vi "CPP-BLplotter.vi"(0 "Plot Array":cluster{dbl[], dbl[]}[](array[cluster])=[{[500.0, 500.0, 953.54, 215.0, 270.0, 320.0, 445.0, 525.0, 600.0, 675.0, 750.0, 825.0, 900.0, 960.0, 1010.0, 1060.0], [4.614524, 4.54365, 5.818368, 0.1374656, 0.6662545, 1.465458, 3.619824, 4.848976, 5.887329, 5.940571, 6.152151, 5.717487, 5.600293, 5.40069, 5.154843, 5.121789]}, {[100.0, 150.0, 215.0, 270.0, 320.0, 445.0, 525.0, 600.0, 675.0, 750.0, 825.0, 900.0, 960.0, 1010.0, 1060.0], [0.002314715, -0.00693192, 0.120417, 0.6880509, 1.519176, 3.513709, 5.065183, 6.116033, 6.096773, 5.938465, 5.593788, 5.5597, 5.387002, 5.304077, 4.887903]}] {"?" format="%.2f"; "?" format="%.2f"}, 1 "Job Directory":path=path "/G4_2_HD/Users/paulhayden/Documents/Projects/Westlakes_resolution") -> (2 "Saved Automatically?":bool, 3 "gnuplotScript":string="set term epslatex\nset output \"Plot.eps\"\nset xlabel '$Distance~(m)$'\nset ylabel '$DF~(s/m^3)\\times10^6$'\nset samples 1000\nset pointsize 1.00\nset title '$B38~Centreline~Glc$' 0, 0\nset size 0.75,0.9\n\n#set key 450, -2.5833\n unset key\nset label 1 '~~~~~~~~~~~Angle~(deg)~=~0' at -100, -2.58\nset label 2 '~~~~~~~~~~~Height~(m)~=~5' at -100, -3.27\n set xrange [0 : 500] \n# set autoscale x \n set yrange [0.10000 : 7]\n# set autoscale y \n\nplot \"B38_Centreline_Glc.dat\" index 0 using 1:2 axes x1y1 title '$File=B38R~DDD.xls$' with points 1 1, \\\n\"B38_Centreline_Glc.dat\" index 1 using 1:2 axes x1y1 title '$File=B38R~DDD~1.xls$' with points 1 3", 4 "Plot data file":path)   [LabVIEW 2012]
uses:
  Results_plotter_Global.vi
panel:
  in  "Tab Control":enum32{"Good Shit", "Boring Shit"}(tab)
  in  "Cancel Button":bool
  in  "Print Button":bool
  out "Velocity":cluster{dbl[], dbl[]}(graph)
  out "Turbulence":cluster{dbl[], dbl[]}(graph)
  in  "Plot Title":u16(ring) items=["Title String Only", "Number of Measurements", "Date::", "Profile::", "Multi Run:Start Time:", "Multi Run:Row:Type", "Multi Run:Row:Number", "Point:Time:", "Time:Stamp:", "Measuring:Instrument:Type", "Multirun:Comments:", "Run:Messages:", "Repeat::", "U_{HF}/U_{ref}::", "U_{5HP}/U_{ref}::", "TI_{HF}:%:", "TI_{U(5HP)}:%:", "Vmag_{5HP}/U_{ref}::", "V_{5HP}/U_{5HP}::", "W_{5HP}/U_{5HP}::", "U_{ref}::", "U_{HF}::", "Vmag_{5HP}::", "U_{5HP}::", "V_{5HP}::", "W_{5HP}::", "L(U):Est:(m)", "X_{5HP}:(mm):", "X_{HF}:(mm):", "Y_{5HP}:(mm):", "Y_{HF}:(mm):", "Z_{5HP}:(mm):", "Z_{HF}:(mm):", "Tau(HF)::", "Tau(5HP1)::(nose)", "Tau(5HP2)::(bottom)", "Tau(5HP3)::(top)", "Tau(5HP4)::(side)", "Tau(5HP5)::(side)", "uhf^2::", "uhf^3/(uhf^2)^1.5::", "(uhf^4/(uhf^2)^2) -3::", "HW (Uhf):Standard Error:in Mean", "HW (Uhf):Standard Error:in Variance", "HW (Uhf):Calibration:Filename", "5HP:Mode:", "5HP:ReturnType:", "Reference:Temperature:Used for Corrections", "Atmos:Pressure:Used for Corrections", "Av Analogue:Sampling:Rate", "No of:Analogue:Samples", "No Of:Measurement:Blocks", "Flow:Measurement:Time", "X:(URef):(mm)", "Y:(URef):(mm)", "Z:(URef):(mm)", "Original:Results:Filename", "Current:Data:Filename", "Current:Data File:1st Folder level", "Current:Data File:2nd Folder level", "Current:Data File:3rd Folder level", "Current:Data File:4th Folder level", "Current:File:Number", "Raw:Data:Filename", "Tunnel1 Metadata:Profile:Code", "Vmag_SD::", "U_SD::", "V_SD::", "W_SD::", "GoodFraction::"]
  in  "Filename Max length":i32=255
  out "Final Title":string="B38 Centreline Glc"
  out "Path":path
  in  "Plot Title Post Block":string
  in  "Plot Title Pre Block":string
  in  "Show Script Editor?":bool
  out "Array":string[](array[string])
  out "t":string
  # "put a load of nice controls here for ref height etc, then a button to say \"print it\" that makes and runs a gnuplot script for \nthe graphs as you have them....."
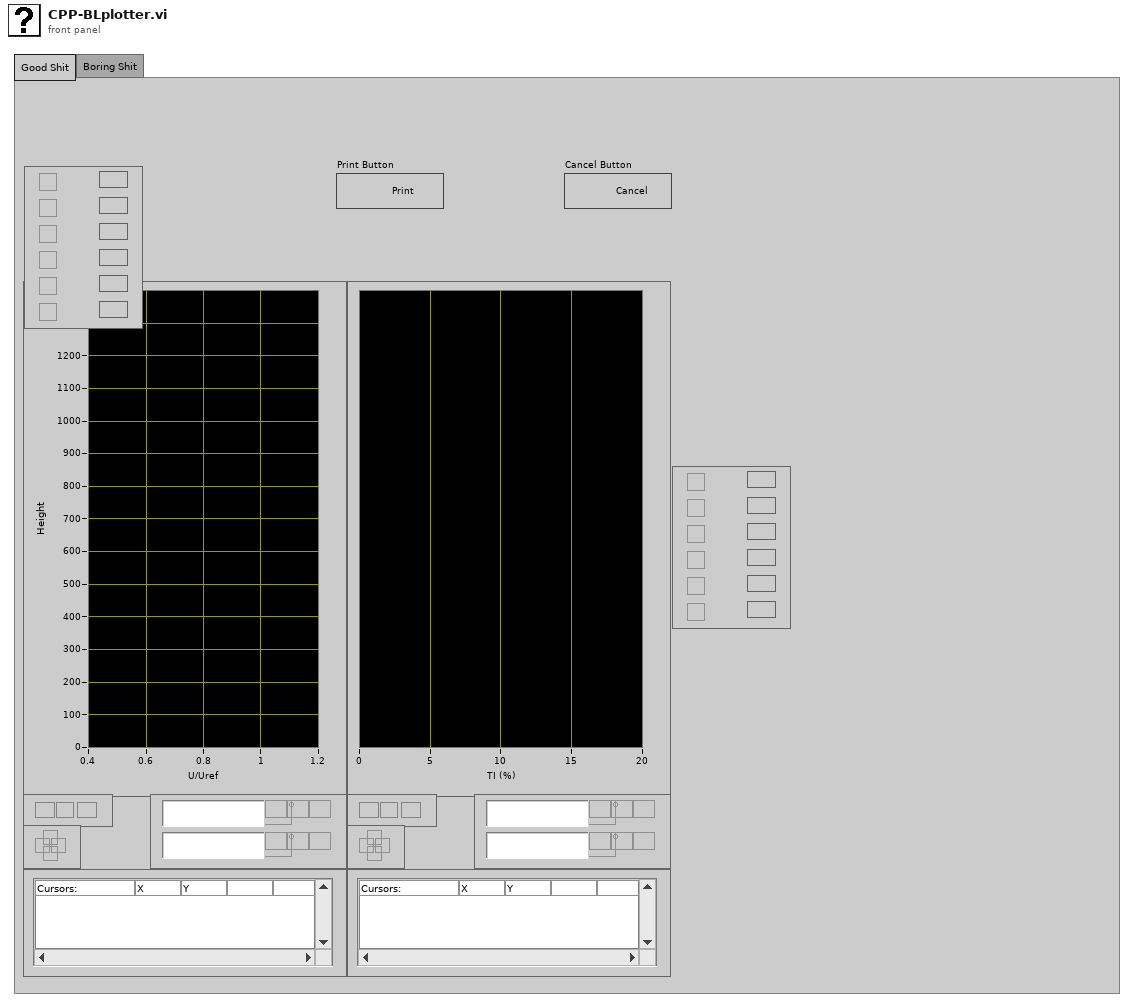
[diagram p1: front panel]
types:
  T1 = typedef "LVRangeTypeDef.ctl" = cluster{"Minimum":dbl, "Maximum":dbl, "Increment":dbl, "Minor Increment":dbl, "Start":dbl}
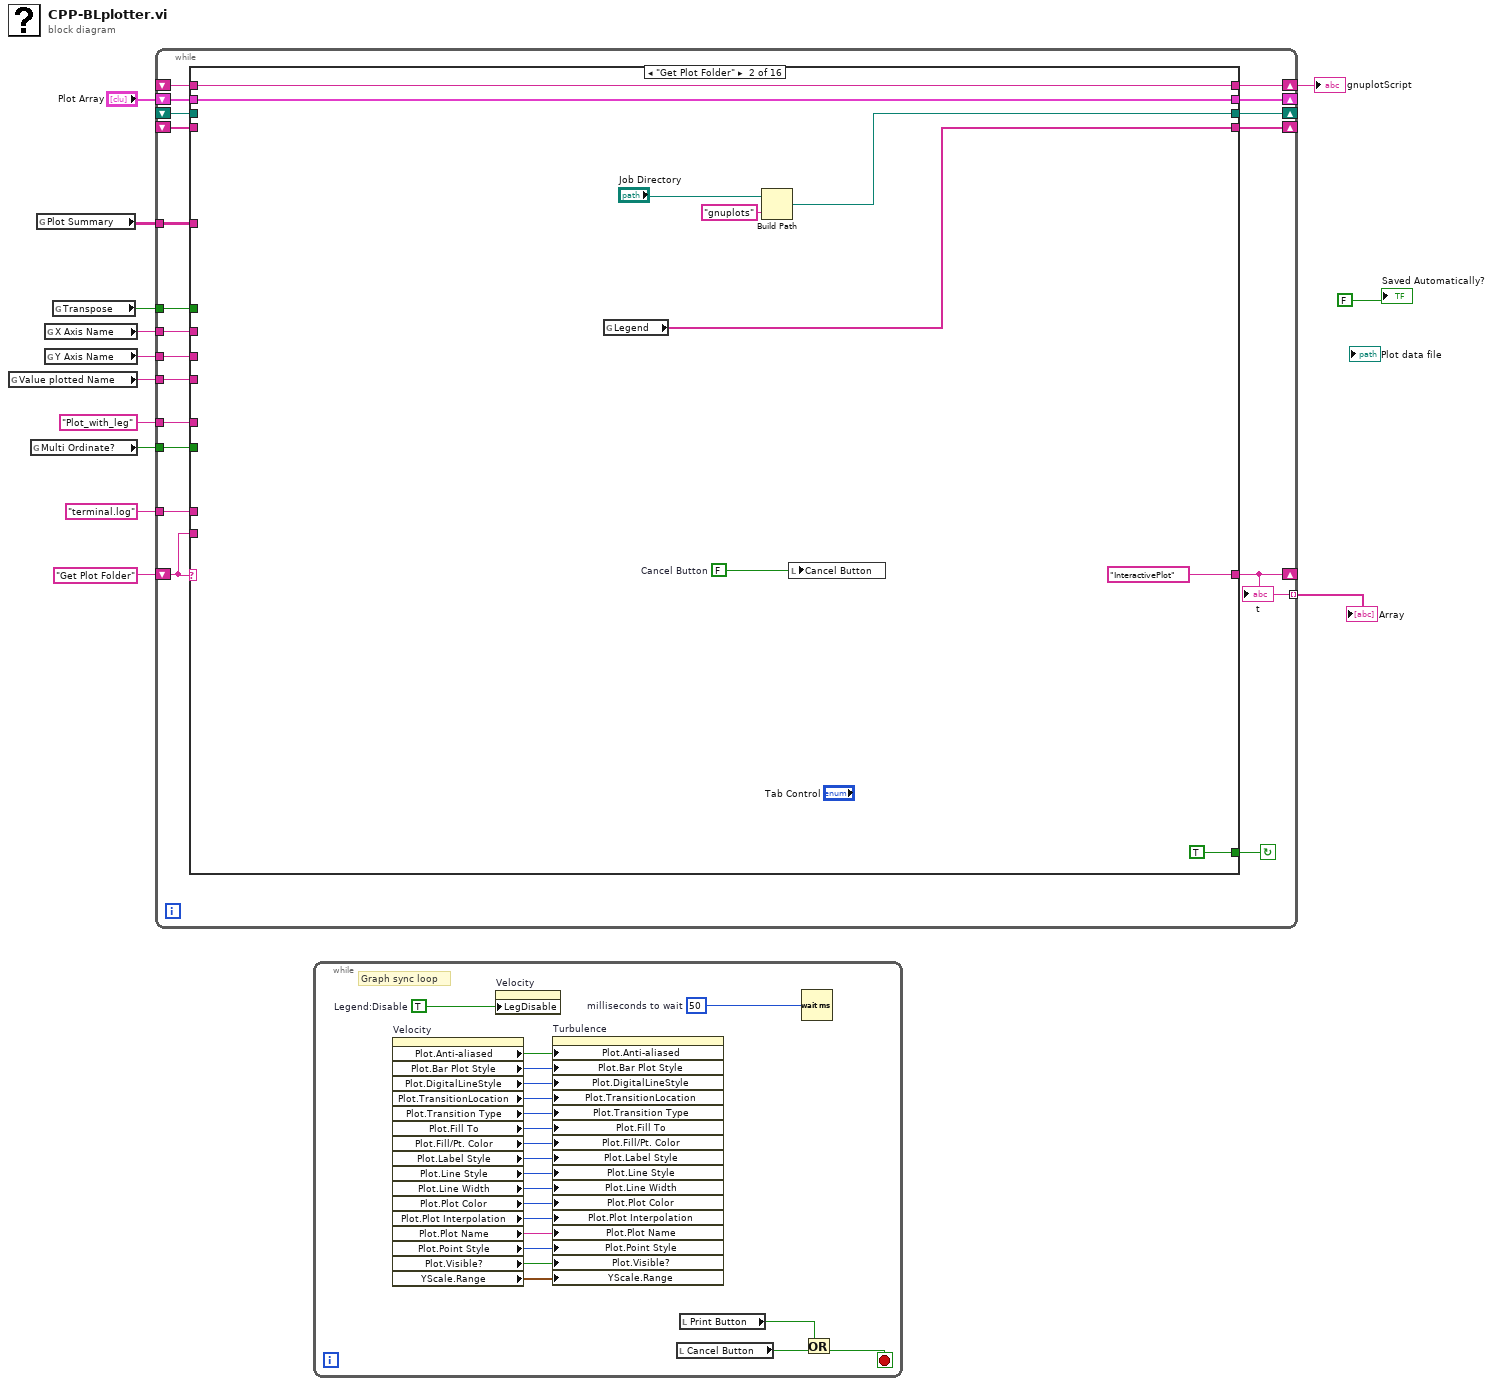
[diagram p0: block diagram]
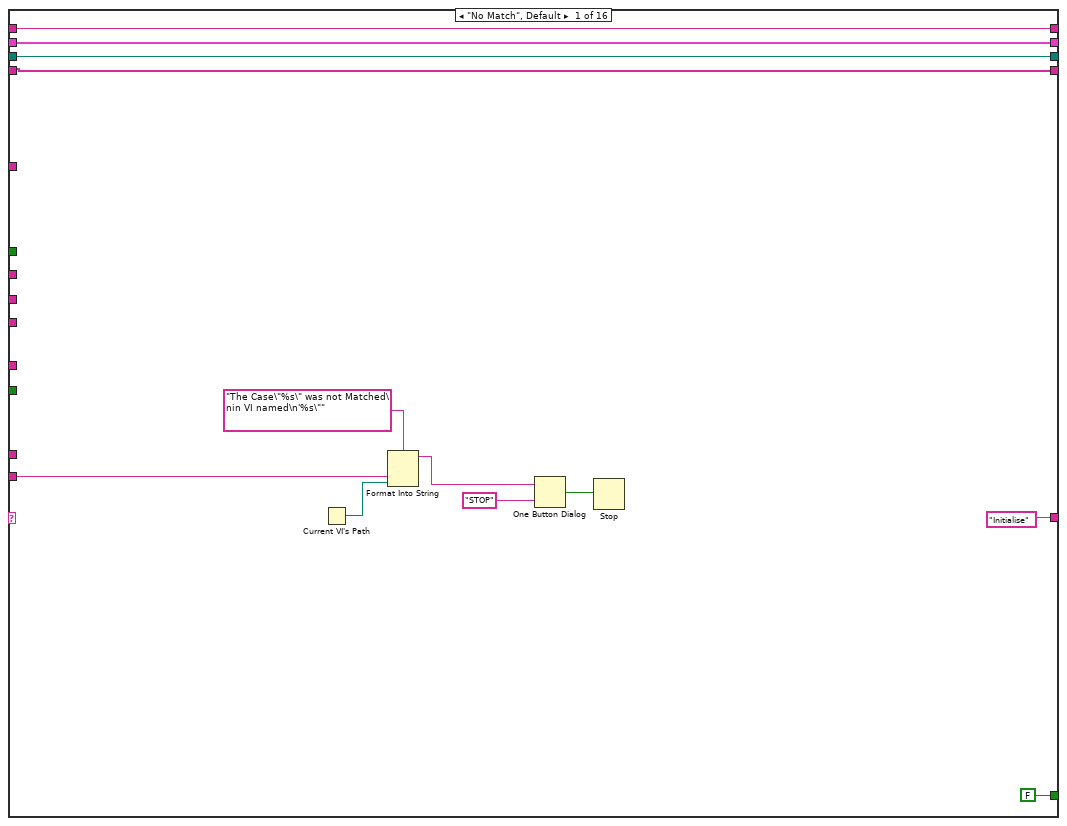
[diagram p2: hidden frame]
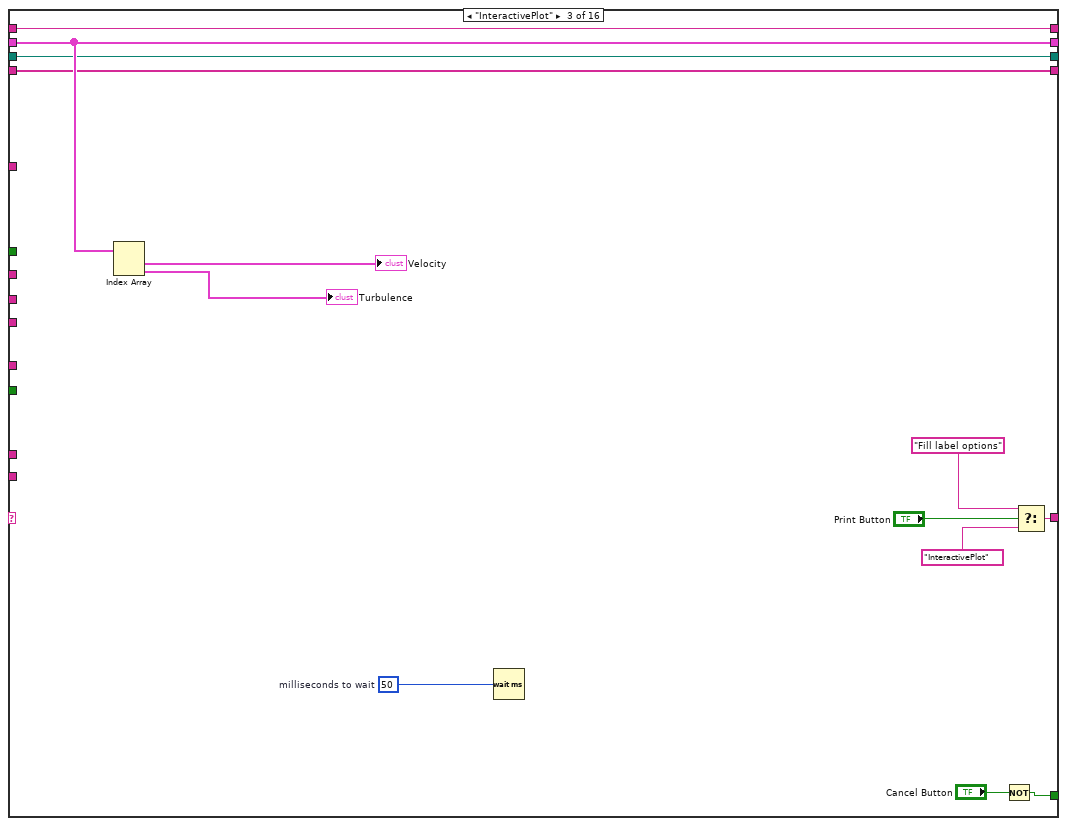
[diagram p3: hidden frame]
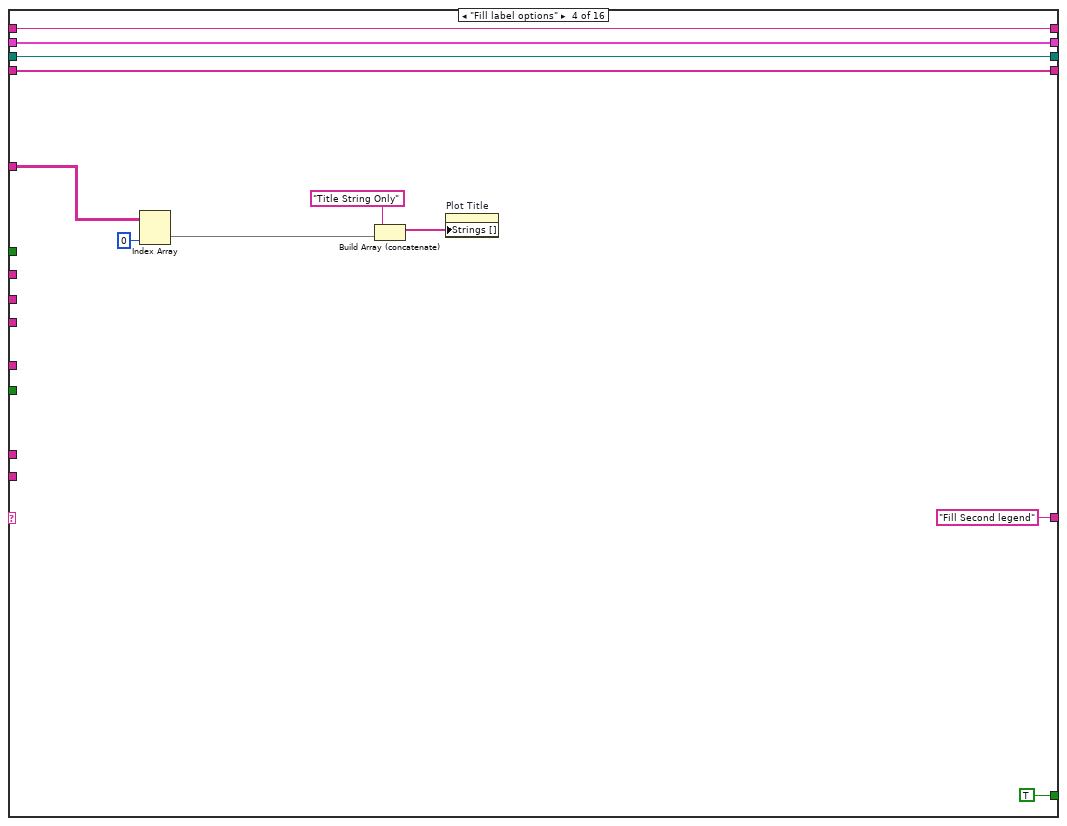
[diagram p4: hidden frame]
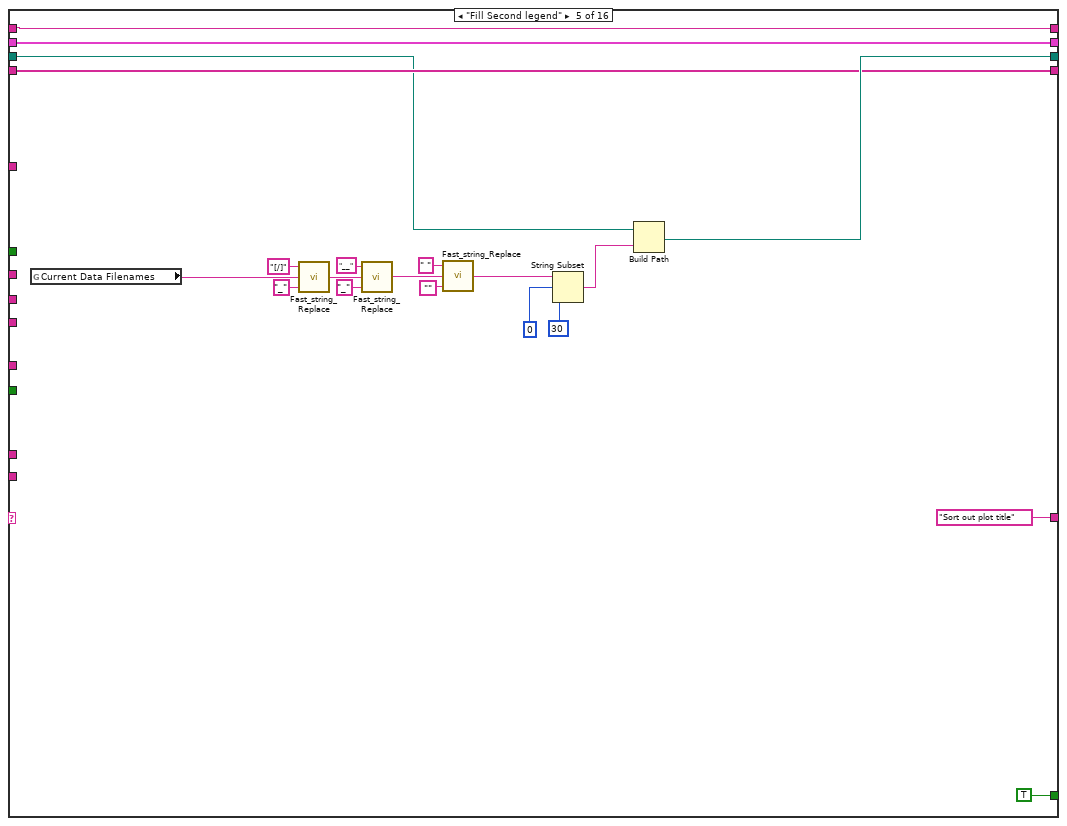
[diagram p5: hidden frame]
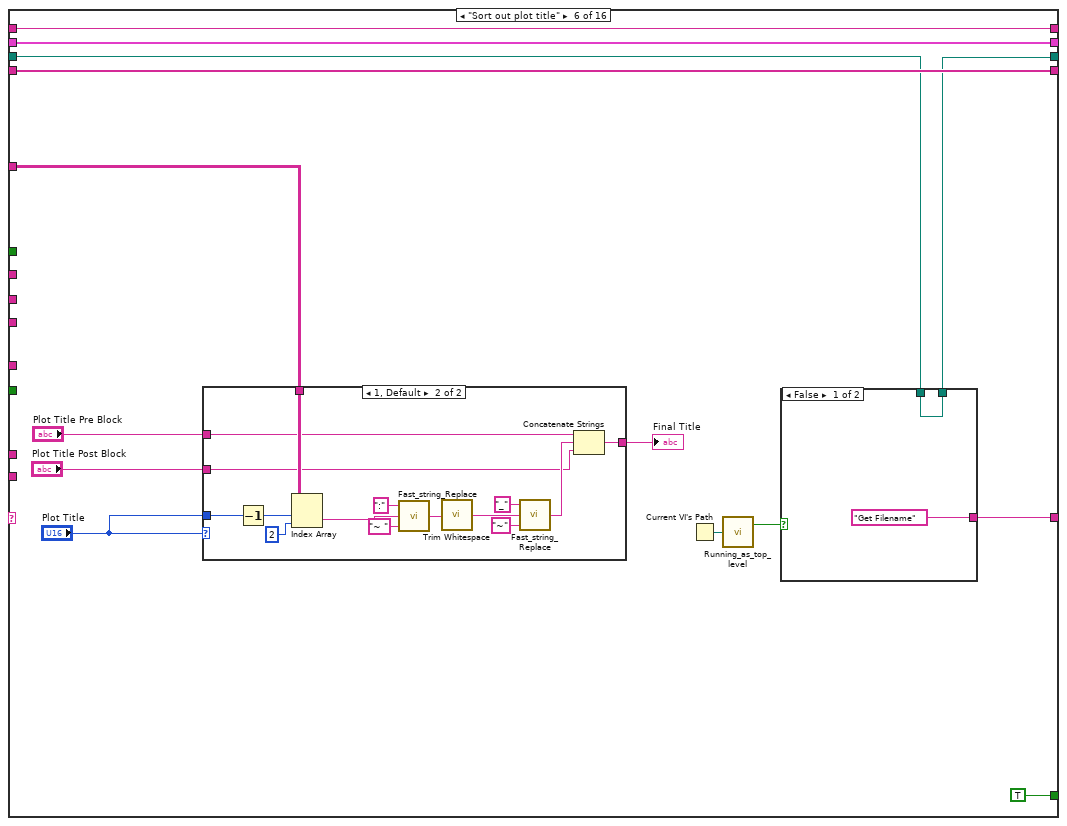
[diagram p6: hidden frame]
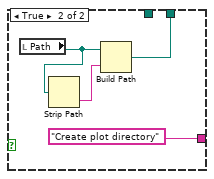
[diagram p7: hidden frame]
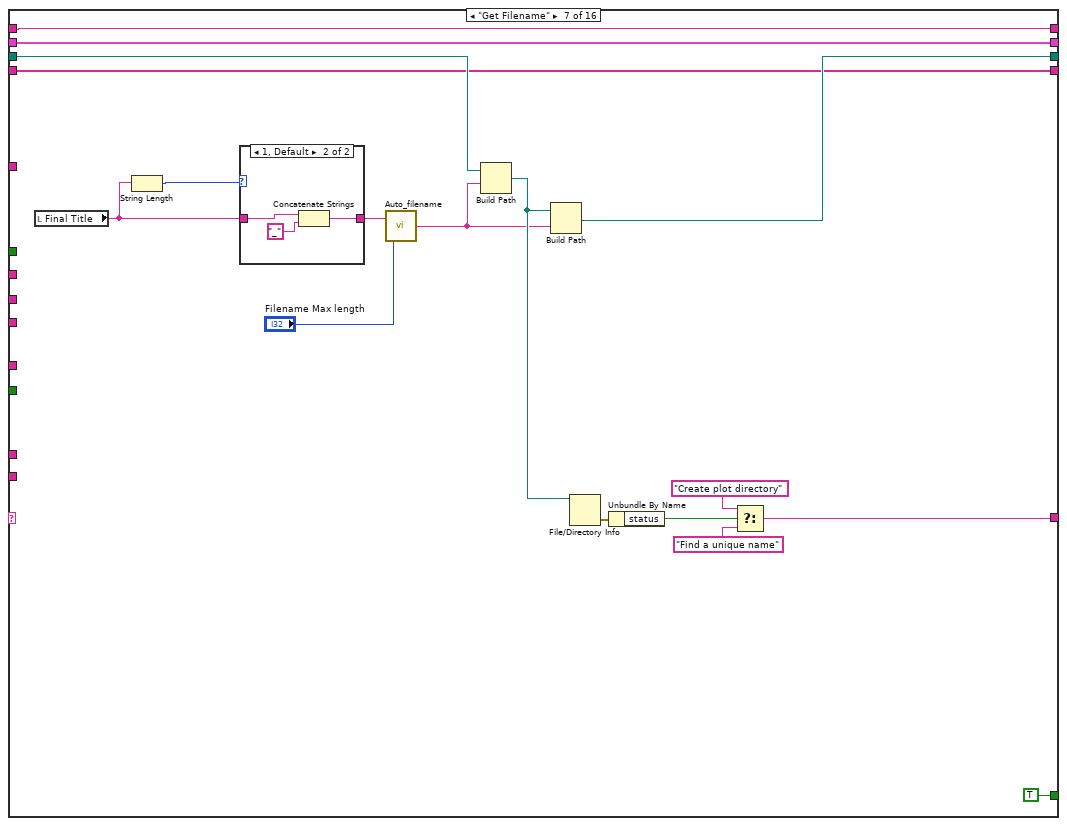
[diagram p9: hidden frame]
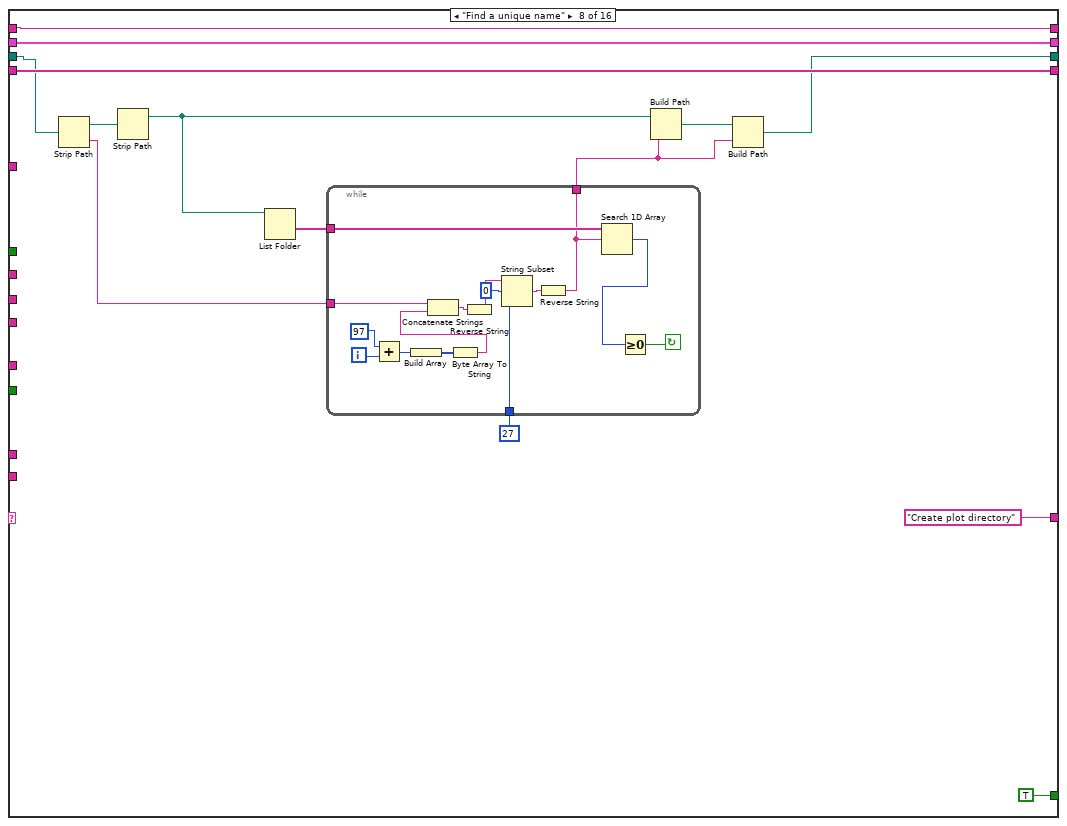
[diagram p11: hidden frame]
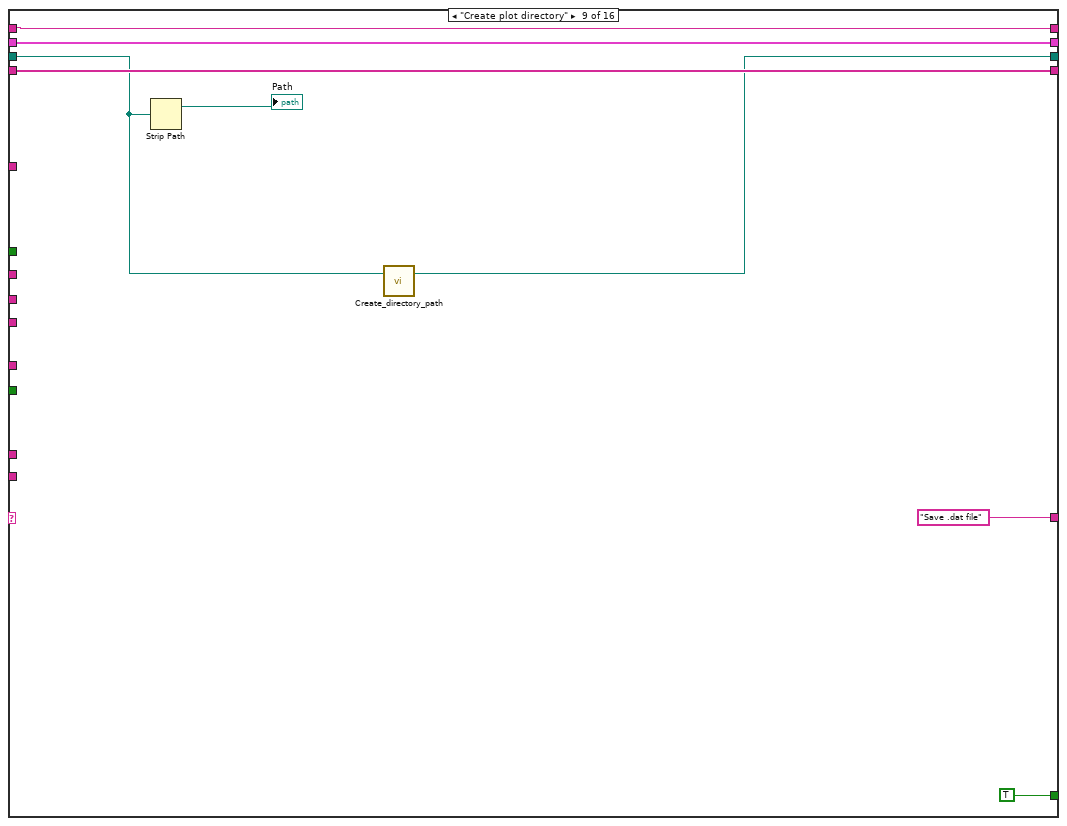
[diagram p12: hidden frame]
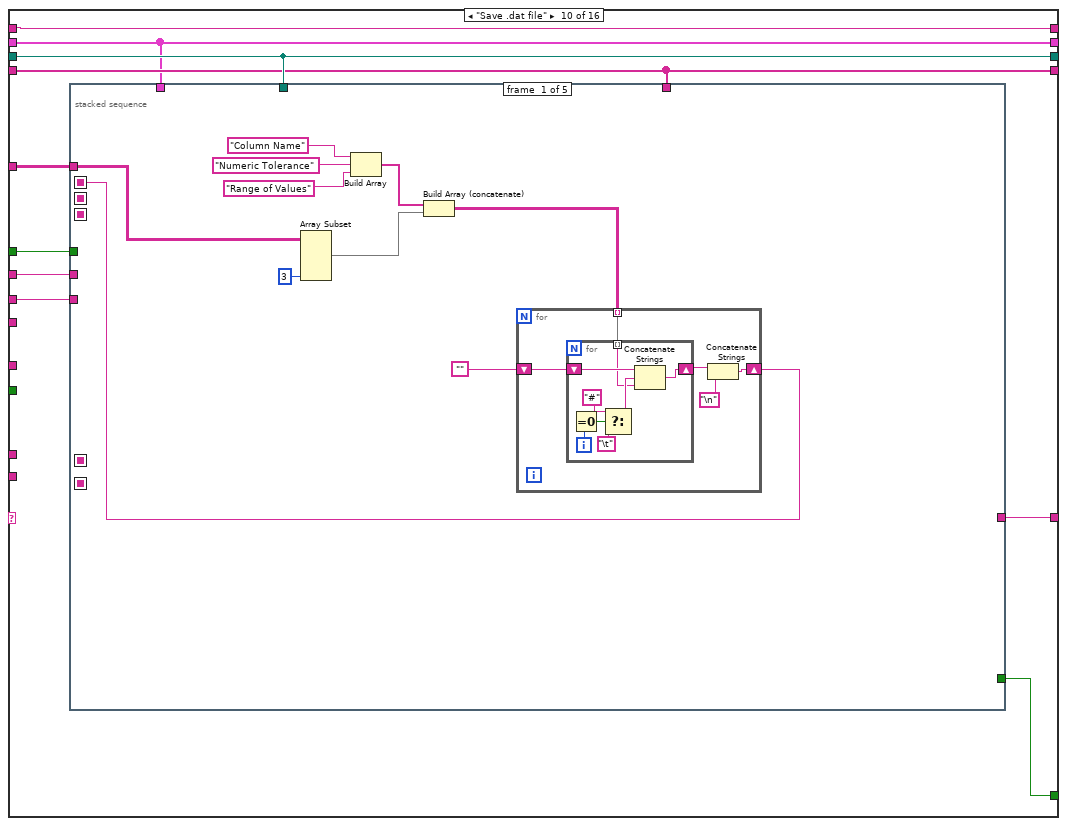
[diagram p13: hidden frame]
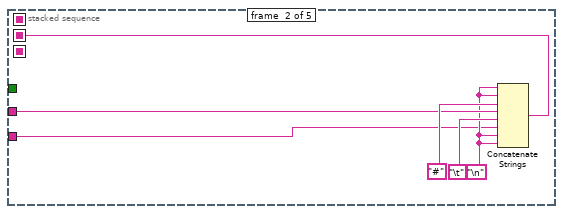
[diagram p14: hidden frame]
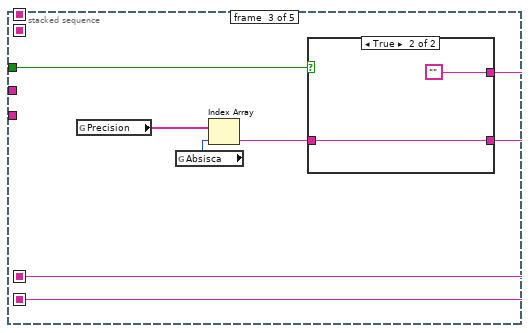
[diagram p15: hidden frame]
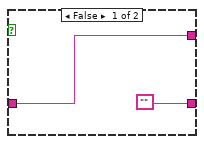
[diagram p16: hidden frame]
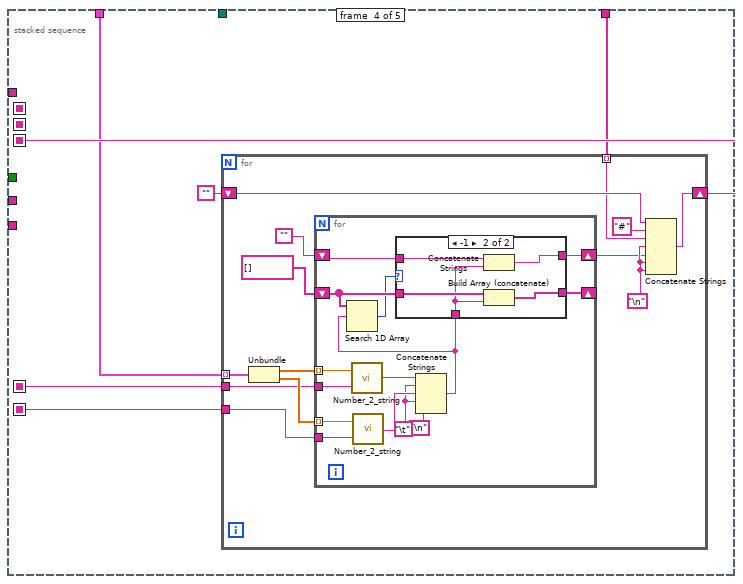
[diagram p17: hidden frame]
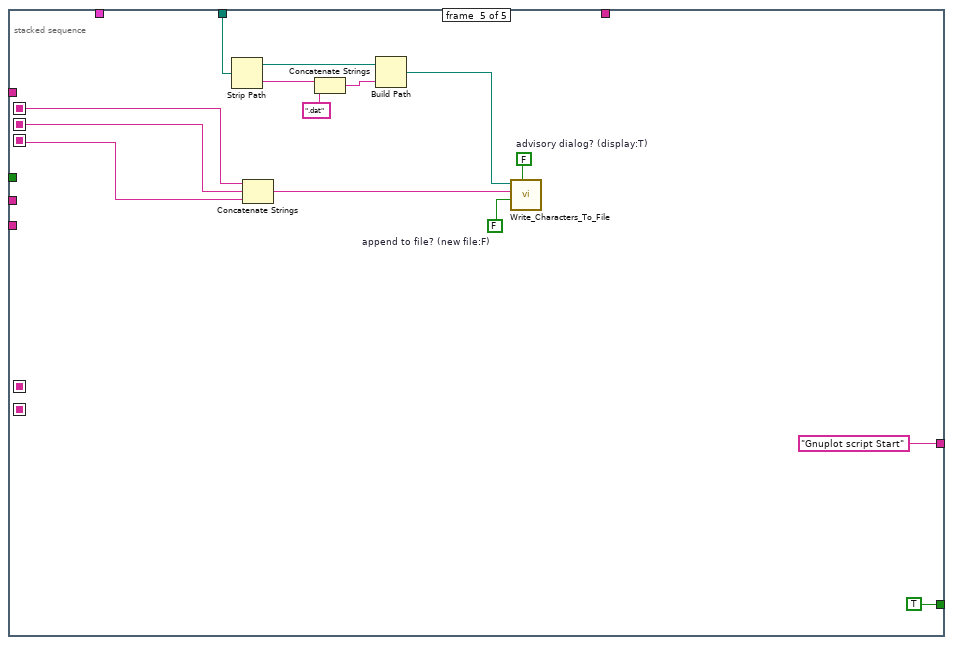
[diagram p19: hidden frame]
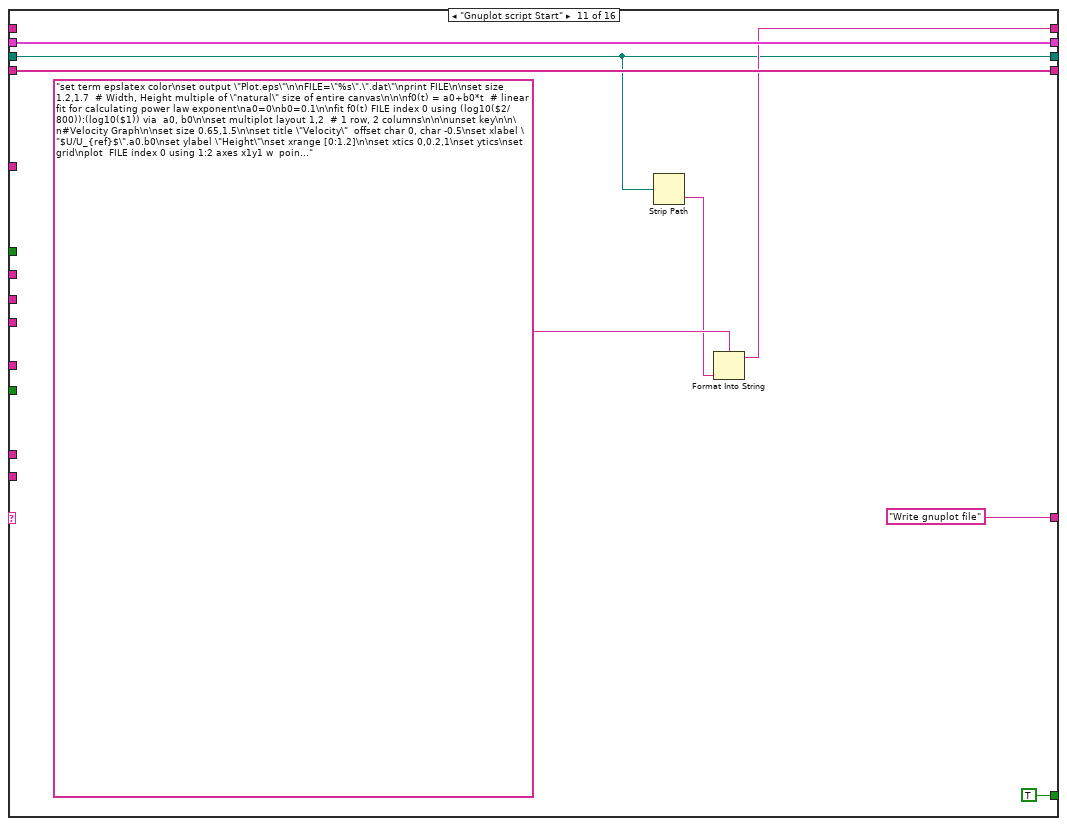
[diagram p20: hidden frame]
diagram:
  n1 = global read "Results_plotter_Global.vi" "Value plotted Name"() -> (w9:string)
  n2 = global read "Results_plotter_Global.vi" "Multi Ordinate?"() -> (w2:bool)
  n3 = global read "Results_plotter_Global.vi" "Plot Summary"() -> (w12:string[][])
  n4 = global read "Results_plotter_Global.vi" "X Axis Name"() -> (w11:string)
  n5 = global read "Results_plotter_Global.vi" "Y Axis Name"() -> (w10:string)
  n6 = global read "Results_plotter_Global.vi" "Transpose"() -> (w3:bool)
  n7 = while {
    shift-left: "Get Plot Folder" -> [w31]
    shift-right: [w14] -> _
    tunnel: w12 -> [w30]
    shift-right: [w29] -> _
    shift-left: _ -> [w28]
    tunnel: w11 -> [w27]
    tunnel: w10 -> [w26]
    tunnel: w9 -> [w25]
    shift-right: [w23] -> _
    shift-left: "Plot Array" -> [w24]
    shift-right: [w21] -> w8
    shift-left: _ -> [w22]
    tunnel: "Plot_with_leg" ("name or relative path") -> [w20]
    shift-right: [w19] -> _
    shift-left: _ -> [w18]
    tunnel: "terminal.log" -> [w17]
    tunnel: w3 -> [w16]
    tunnel: w2 -> [w15]
    tunnel: [w14] -> w1 mode=indexing
    stop <- w32 continue-if-true
    n8 = case shown="\"Get Plot Folder\"" w31 {
      tunnel: [FALSE TRUE w55 TRUE ("Top Level") TRUE ("Top Level") TRUE ("Top Level") TRUE ("Top Level") TRUE ("Top Level") TRUE w199 TRUE ("Top Level") TRUE ("Top Level") TRUE ("Top Level") TRUE ("Top Level") FALSE ("Top Level") FALSE ("Top Level")] -> w32
      tunnel: ["Initialise" "InteractivePlot" w60 "Fill Second legend" "Sort out plot title" w99 w148 "Create plot directory" "Save .dat file" w198 "Write gnuplot file" ("t") "Execute shell script" ("t") "Has pdf been generated?" ("t") w322 "End" "End" ("t")] -> w14
      tunnel: w31 -> [w39 _ _ _ _ _ _ _ _ _ _ _ _ _ _ _]
      tunnel: w30 -> [_ _ _ w77 _ w106 _ _ _ w197 _ _ _ _ _ _]
      tunnel: [w36 w50 w63 w71 w97 w101 w149 w155 w188 w200 w297 w307 w315 w326 w331 w341] -> w29
      tunnel: w28 -> [w36 _ w63 w71 w93 w100 w145 w162 w187 w200 w297 w307 w315 w326 w331 w341]
      tunnel: w27 -> [_ _ _ _ _ _ _ _ _ w196 _ _ _ _ _ _]
      tunnel: w26 -> [_ _ _ _ _ _ _ _ _ w195 _ _ _ _ _ _]
      tunnel: w25 -> [_ _ _ _ _ _ _ _ _ _ _ _ _ _ _ _]
      tunnel: w24 -> [w35 w47 w64 w72 w96 w111 w147 w165 w191 w192 w302 w313 w320 w329 w336 w346]
      tunnel: [w35 w47 w64 w72 w96 w111 w147 w165 w191 w192 w302 w313 w320 w329 w336 w346] -> w23
      tunnel: w22 -> [w34 w49 w61 w73 w95 w107 w146 w164 w190 w201 _ w303 w318 w327 w334 w344]
      tunnel: [w34 w49 w61 w73 w95 w107 w146 w164 w190 w201 w298 w303 w318 w327 w334 w344] -> w21
      tunnel: w20 -> [_ _ _ _ _ _ _ _ _ _ _ _ _ _ _ _]
      tunnel: [w33 w46 w62 w70 w94 w110 w144 w163 w189 w194 w301 w308 w319 w328 w335 w345] -> w19
      tunnel: w18 -> [w33 _ w62 w70 w94 w110 w144 w163 w189 w194 w301 w308 w319 w328 w335 w345]
      tunnel: w17 -> [_ _ _ _ _ _ _ _ _ _ _ _ w314 _ _ w339]
      tunnel: w16 -> [_ _ _ _ _ _ _ _ _ w193 _ _ _ _ _ _]
      tunnel: w15 -> [_ _ _ _ _ _ _ _ _ _ _ _ _ _ _ _]
      frame "No Match", Default {
        n9 = Current VI's Path() -> (path=w38:path)
        n10 = Format Into String(format string="The Case\"%s\" was not Matched\nin VI named\n'%s\"" ("Format String"), w39, w38) -> (resulting string=w42:string)  [unwired: 2 in, 1 out]
        n11 = One Button Dialog(message=w42, button name ("OK")="STOP") -> (true=w40:bool)
        n12 = Stop(stop? (T)=w40) -> ()
      }
      frame "Get Plot Folder" {
        w45 = FALSE  # Cancel Button
        n13 = global read "Results_plotter_Global.vi" "Legend"() -> (w46:string[])
        n14 = Build Path(base path="Job Directory", name or relative path="gnuplots") -> (appended path=w50:path)
        n15 = local write "Cancel Button"(w45) -> ()
      }
      frame "InteractivePlot" {
        w54 = u32 50  # milliseconds to wait
        n16 = Index Array(array=w64) -> (element #1=→"Velocity":cluster{dbl[], dbl[]}, element #2=→"Turbulence":cluster{dbl[], dbl[]})  [unwired: 2 in]
        n17 = Wait (ms)(milliseconds to wait=w54) -> ()  [unwired: 1 out]
        n18 = Not(x="Cancel Button") -> (.not. x?=w55:bool)
        n19 = Select(t="Fill label options", s="Print Button", f="InteractivePlot") -> (s? t:f=w60:string)
      }
      frame "Fill label options" {
        n20 = Index Array(array=w77, index (col)=0 ("disabled index (col)")) -> (element=w68:string[])  [unwired: 1 in]
        n21 = Build Array (concatenate)("Title String Only", w68) -> (w67:string[])
        n22 = property on="Plot Title" class="Ring (strict)"("Strings []"=w67) -> ()  [unwired: 2 in, 2 out]
      }
      frame "Fill Second legend" {
        n23 = global read "Results_plotter_Global.vi" "Current Data Filenames"() -> (w82:string)
        n24 = call "Fast_string_Replace.vi"("Replace match with:"="_", "Input String"=w82, "regular expression"="[/]") -> ("Output String"=w86:string)  [unwired: 2 out]
        n25 = call "Fast_string_Replace.vi"("Replace match with:"="_", "Input String"=w86, "regular expression"="__") -> ("Output String"=w83:string)  [unwired: 2 out]
        n26 = call "Fast_string_Replace.vi"("Replace match with:"="", "Input String"=w83, "regular expression"=" ") -> ("Output String"=w81:string)  [unwired: 2 out]
        n27 = String Subset(string=w81, offset (0)=0, length (rest)=30 ("length (rest)")) -> (substring=w80:string)
        n28 = Build Path(base path=w93, name or relative path=w80) -> (appended path=w97:path)
      }
      frame "Sort out plot title" {
        n29 = case shown="1, Default" "Plot Title" {
          tunnel: [w118 w123] -> w105
          tunnel: "Plot Title Pre Block" -> [w118 w122]
          tunnel: w106 -> [_ w126]
          tunnel: "Plot Title" -> [_ w125]
          tunnel: "Plot Title Post Block" -> [_ w119]
          frame 0 {
          }
          frame 1, Default {
            n30 = Decrement(x=w125) -> (x-1=w124:u16)
            n31 = Index Array(array=w126, index (row)=w124, index (col)=u16 2 ("y")) -> (element=w129:string)
            n32 = call "Fast_string_Replace.vi"("Replace match with:"="~ ", "Input String"=w129, "regular expression"=":") -> ("Output String"=w128:string)  [unwired: 2 out]
            n33 = call <vilib>:"Trim Whitespace.vi"("string"=w128) -> ("trimmed string"=w127:string)  [unwired: 1 in]
            n34 = call "Fast_string_Replace.vi"("Replace match with:"="~", "Input String"=w127, "regular expression"="_") -> ("Output String"=w121:string)  [unwired: 2 out]
            n35 = Concatenate Strings(w122, w121, w119) -> (w123:string)
          }
        }
        "Final Title" <- w105
        n36 = Current VI's Path() -> (path=w104:path)
        n37 = call "Running_as_top_level.vi"("Vi path name"=w104) -> ("Top Level"=w102:bool)  [unwired: 1 out]
        n38 = case shown="False" w102 {
          tunnel: [w113 w116] -> w101
          tunnel: w100 -> [w113 _]
          tunnel: ["Get Filename" ("t") "Create plot directory"] -> w99
          frame False {
          }
          frame True {
            n39 = local read "Path"() -> (w115:path)
            n40 = Strip Path(path=w115) -> (name=w114:string)  [unwired: 1 out]
            n41 = Build Path(base path=w115, name or relative path=w114) -> (appended path=w116:path)
          }
        }
      }
      frame "Get Filename" {
        n42 = local read "Final Title"() -> (w134:string)
        n43 = String Length(string=w134) -> (length=w136:i32)
        n44 = case shown="1, Default" w136 {
          tunnel: [w151 w152] -> w135
          tunnel: w134 -> [w151 w154]
          frame 0 {
          }
          frame 1, Default {
            n45 = Concatenate Strings(w154, "_") -> (w152:string)
          }
        }
        n46 = call "Auto_filename.vi"("Filename Max length"="Filename Max length", "Prefix"=w135) -> ("Filename"=w138:string)
        n47 = Build Path(base path=w145, name or relative path=w138) -> (appended path=w142:path)
        n48 = Build Path(base path=w142, name or relative path=w138) -> (appended path=w149:path)
        n49 = File/Directory Info(path=w142) -> (error out=w143:errorcluster)  [unwired: 1 in, 6 out]
        n50 = Unbundle By Name(w143) -> ("status"=w141:bool)
        n51 = Select(t="Create plot directory", s=w141, f="Find a unique name") -> (s? t:f=w148:string)
      }
      frame "Find a unique name" {
        n52 = Strip Path(path=w162) -> (stripped path=w161:path, name=w160:string)
        n53 = Strip Path(path=w161) -> (stripped path=w158:path)  [unwired: 1 out]
        n54 = List Folder(path=w158) -> (folder names=w159:string[])  [unwired: 1 in, 5 out]
        n55 = while {
          tunnel: w160 -> [w183]
          tunnel: 27 ("Max Length") -> [w182]
          tunnel: [w171] -> w157
          tunnel: w159 -> [w172]
          i -> [w173]
          stop <- w169 continue-if-true
          n56 = Add(x=97, y=w173) -> (x+y=w180:i32)
          n57 = Build Array(w180) -> (w181:i32[])
          n58 = Byte Array To String(unsigned byte array=w181) -> (string=w178:string)
          n59 = Concatenate Strings(w183, w178) -> (w176:string)
          n60 = Reverse String(1:w176) -> (0:w177:string)
          n61 = String Subset(string=w177, offset (0)=0, length (rest)=w182) -> (substring=w175:string)
          n62 = Reverse String(1:w175) -> (0:w171:string)
          n63 = Search 1D Array(1D array=w172, element=w171) -> (index of element=w170:i32)  [unwired: 1 out]
          n64 = Greater Or Equal To 0?(x=w170) -> (x >= 0?=w169:bool)
        }
        n65 = Build Path(base path=w158, name or relative path=w157) -> (appended path=w156:path)
        n66 = Build Path(base path=w156, name or relative path=w157) -> (appended path=w155:path)
      }
      frame "Create plot directory" {
        n67 = Strip Path(path=w187) -> (stripped path=→"Path":path)  [unwired: 1 out]
        n68 = call "Create_directory_path.vi"("Path name"=w187) -> ("Path name Out"=w188:path)  [unwired: 1 in, 1 out]
      }
      frame "Save .dat file" {
        n69 = stacked-sequence {
          seq-local: [w202 _ _ _ _] -> [_ _ _ _ w286]
          seq-local: [_ w226 _ _ _] -> [_ _ _ _ w287]
          seq-local: [_ _ _ w245 _] -> [_ _ _ _ w288]
          seq-local: [_ _ w231 _ _] -> [_ _ _ w243 _]
          seq-local: [_ _ w233 _ _] -> [_ _ _ w242 _]
          tunnel: w200 -> [_ _ _ _ w291]
          tunnel: [_ _ _ _ TRUE ("Top Level")] -> w199
          tunnel: [_ _ _ _ "Gnuplot script Start"] -> w198
          tunnel: w197 -> [w207 _ _ _ _]
          tunnel: w196 -> [_ w229 _ _ _]
          tunnel: w195 -> [_ w225 _ _ _]
          tunnel: w192 -> [_ _ _ w241 _]
          tunnel: w194 -> [_ _ _ w244 _]
          tunnel: w193 -> [_ _ w234 _ _]
          frame #0 {
            n70 = Array Subset(array=w207, length (col)=3 ("length")) -> (w205:string[][])  [unwired: 3 in]
            n71 = Build Array("Column Name", "Numeric Tolerance", "Range of Values") -> (w211:string[])
            n72 = Build Array (concatenate)(w211, w205) -> (w203:string[][])
            n73 = for {
              shift-right: [w215] -> w202
              shift-left: "" -> [w212]
              tunnel: w203 -> [w216] mode=indexing
              n74 = for {
                shift-right: [w217] -> w214
                shift-left: w212 -> [w224]
                tunnel: w216 -> [w218] mode=indexing
                i -> [w223]
                n75 = Equal To 0?(x=w223) -> (x = 0?=w222:bool)
                n76 = Select(t="#", s=w222, f="\t") -> (s? t:f=w219:string)
                n77 = Concatenate Strings(w224, w219, w218) -> (w217:string)
              }
              n78 = Concatenate Strings(w214, "\n") -> (w215:string)
            }
          }
          frame #1 {
            w227 = "\n"
            n79 = Concatenate Strings(w227, w227, "#" ("string"), w229, "\t", w225, w227, w227) -> (w226:string)
          }
          frame #2 {
            n80 = global read "Results_plotter_Global.vi" "Precision"() -> (w236:string[])
            n81 = global read "Results_plotter_Global.vi" "Absisca"() -> (w235:i32)
            n82 = Index Array(array=w236, index=w235) -> (element=w232:string)
            n83 = case shown="True" w234 {
              tunnel: ["" w240] -> w233
              tunnel: w232 -> [w237 w240]
              tunnel: [w237 ""] -> w231
              frame False {
              }
              frame True {
              }
            }
          }
          frame #3 {
            n84 = for {
              tunnel: w241 -> [w259] mode=indexing
              shift-right: [w258] -> w245
              shift-left: "" -> [w252]
              tunnel: w244 -> [w250] mode=indexing
              tunnel: w243 -> [w248]
              tunnel: w242 -> [w247]
              w257 = "\n"
              n85 = Unbundle(w259) -> (w253:dbl[], w254:dbl[])
              n86 = for {
                tunnel: w253 -> [w273] mode=indexing
                shift-right: [w268] -> w256
                shift-left: "" -> [w269]
                tunnel: w254 -> [w261] mode=indexing
                shift-right: [w267] -> _
                shift-left: string[] [] -> [w266]
                tunnel: w248 -> [w263]
                tunnel: w247 -> [w262]
                w270 = "\t"
                n87 = call "Number_2_string.vi"("precision"=w263, "number"=w273) -> ("String"=w272:string)
                n88 = call "Number_2_string.vi"("precision"=w262, "number"=w261) -> ("String"=w271:string)
                n89 = Concatenate Strings(w272, w270, w271, w270, "\n") -> (w265:string)
                n90 = Search 1D Array(1D array=w266, element=w265) -> (index of element=w264:i32)  [unwired: 1 in]
                n91 = case shown="-1" w264 {
                  tunnel: w269 -> [w275 w280]
                  tunnel: [w275 w279] -> w268
                  tunnel: w265 -> [_ w276]
                  tunnel: w266 -> [w274 w278]
                  tunnel: [w274 w277] -> w267
                  frame 0, Default {
                  }
                  frame -1 {
                    n92 = Concatenate Strings(w280, w276) -> (w279:string)
                    n93 = Build Array (concatenate)(w278, w276) -> (w277:string[])
                  }
                }
              }
              n94 = Concatenate Strings(w252, "#", w250, w257, w256, w257, w257) -> (w258:string)
            }
          }
          frame #4 {
            w283 = FALSE  # advisory dialog? (display:T)
            w284 = FALSE  # append to file? (new file:F)
            n95 = Strip Path(path=w291) -> (stripped path=w292:path, name=w294:string)
            n96 = Concatenate Strings(w286, w287, w288) -> (w285:string)
            n97 = Concatenate Strings(w294, ".dat" ("string")) -> (w293:string)
            n98 = Build Path(base path=w292, name or relative path=w293) -> (appended path=w282:path)
            n99 = call "Write_Characters_To_File.vi"("file path (dialog if empty)"=w282, "advisory dialog? (display:T)"=w283, "character string"=w285, "append to file? (new file:F)"=w284) -> ()  [unwired: 1 in, 4 out]
          }
        }
      }
      frame "Gnuplot script Start" {
        n100 = Strip Path(path=w297) -> (name=w295:string)  [unwired: 1 out]
        n101 = Format Into String(format string="set term epslatex color\nset output \"Plot.eps\"\n\nFILE=\"%s\".\".dat\"\nprint FILE\n\nset size 1.2,1.7  # Width, Height multiple of \"natural\" size of entire canvas\n\n\nf0(t) = a0+b0*t  # linear fit for calculating power law exponent\na0=0\nb0=0.1\n\nfit f0(t) FILE index 0 using (log10($2/800)):(log10($1)) via  a0, b0\n\nset multiplot layout 1,2  # 1 row, 2 columns\n\n\nunset key\n\n\n#Velocity Graph\n\nset size 0.65,1.5\n\nset title \"Velocity\"  offset char 0, char -0.5\nset xlabel \"$U/U_{ref}$\".a0.b0\nset ylabel \"Height\"\nset xrange [0:1.2]\n\nset xtics 0,0.2,1\nset ytics\nset grid\nplot  FILE index 0 using 1:2 axes x1y1 w  points lc 0 pointtype 4 pointsize 1, f0(x) w lines\n\n#Turbulence Graph\n\nset size 0.55,1.5\nset origin 0.65,0\n\nset title \"Turbulence\"  offset char 0, char -0.5\nset xlabel \"$TI$\"\nunset ylabel\nset xrange [0:35]\n\nset format y \"\"\nset xtics 5,5\nset ytics\nset grid\nplot  FILE index 1 using 1:2 axes x1y1 w  points lc 1 pointtype 4 pointsize 1\n\n\n\nunset multiplot\n", w295) -> (resulting string=w298:string)  [unwired: 2 in, 1 out]
      }
      frame "Write gnuplot file" {
        w310 = FALSE  # append to file? (new file:F)
        w311 = FALSE  # advisory dialog? (display:T)
        n102 = Strip Path(path=w307) -> (stripped path=w304:path)  [unwired: 1 out]
        n103 = Build Path(base path=w304, name or relative path="gnuplot_script.txt") -> (appended path=w312:path)
        n104 = call "Write_Characters_To_File.vi"("file path (dialog if empty)"=w312, "advisory dialog? (display:T)"=w311, "character string"=w303, "append to file? (new file:F)"=w310) -> ()  [unwired: 1 in, 4 out]
      }
      frame "Execute shell script" {
        n105 = call "Run_Gnuplot_Script.vi"("logfileName"=w314, "workingDirectory"=w315) -> ()
      }
      frame "Has pdf been generated?" {
        n106 = Select(t="Show Re-Run Gnuplot?", s="Show Script Editor?", f="Open Standard output file") -> (s? t:f=w322:string)
      }
      frame "Show Re-Run Gnuplot?" {
        n107 = Strip Path(path=w331) -> (stripped path=w330:path)  [unwired: 1 out]
        n108 = call "Re_run_Gnuplot.vi"("Plot folder (dialog if empty)"=w330) -> ()  [unwired: 4 out]
      }
      frame "Open Standard output file" {
        n109 = Strip Path(path=w341) -> (stripped path=w338:path)  [unwired: 1 out]
        n110 = Format Into String(format string="open \"%s\"", w339) -> (resulting string=w337:string)  [unwired: 2 in, 1 out]
        n111 = call <vilib>:"System Exec.vi"("working directory"=w338, "command line"=w337) -> ()  [unwired: 4 in, 6 out]
      }
    }
    "t" <- w14
  }
  "gnuplotScript" <- w8
  "Array" <- w1
  n112 = while {
    stop <- w350 stop-if-true
    w347 = TRUE  # Legend:Disable
    w348 = u32 50  # milliseconds to wait
    # "Graph sync loop"
    n113 = property on="Velocity" class="XYGraph (strict)"() -> ("Plot.Anti-aliased"=w367:bool, "Plot.Bar Plot Style"=w366:u8, "Plot.DigitalLineStyle"=w365:u8, "Plot.TransitionLocation"=w364:u8, "Plot.Transition Type"=w363:u8, "Plot.Fill To"=w362:i16, "Plot.Fill/Pt. Color"=w361:u32, "Plot.Label Style"=w360:u8, "Plot.Line Style"=w359:u8, "Plot.Line Width"=w358:u8, "Plot.Plot Color"=w357:u32, "Plot.Plot Interpolation"=w356:u8, "Plot.Plot Name"=w355:string, "Plot.Point Style"=w354:u8, "Plot.Visible?"=w353:bool, "YScale.Range"=w352:T1)  [unwired: 2 in, 2 out]
    n114 = property on="Velocity" class="XYGraph (strict)"("LegDisable"=w347) -> ()  [unwired: 2 in, 2 out]
    n115 = property on="Turbulence" class="XYGraph (strict)"("Plot.Anti-aliased"=w367, "Plot.Bar Plot Style"=w366, "Plot.DigitalLineStyle"=w365, "Plot.TransitionLocation"=w364, "Plot.Transition Type"=w363, "Plot.Fill To"=w362, "Plot.Fill/Pt. Color"=w361, "Plot.Label Style"=w360, "Plot.Line Style"=w359, "Plot.Line Width"=w358, "Plot.Plot Color"=w357, "Plot.Plot Interpolation"=w356, "Plot.Plot Name"=w355, "Plot.Point Style"=w354, "Plot.Visible?"=w353, "YScale.Range"=w352) -> ()  [unwired: 2 in, 2 out]
    n116 = local read "Cancel Button"() -> (w351:bool)
    n117 = local read "Print Button"() -> (w349:bool)
    n118 = Wait (ms)(milliseconds to wait=w348) -> ()  [unwired: 1 out]
    n119 = Or(x=w349, y=w351) -> (x .or. y?=w350:bool)
  }
  "Saved Automatically?" <- FALSE
